vi "CH_LM FGV Meter Info.vi"(0 "Meter Index":i32, 2 "Action (read)":T4=enum."read", 5 "Serial Number (\"\")":string, 7 "Meter Info":T1, 11 "error in (no error)":errorcluster) -> (3 "All Meter Indices":i32[](array[numeric]), 4 "Meter Index out":i32, 6 "Serial Number out":string, 8 "Meter Info":T1, 13 "All Serial Numbers":string[](array[string]), 14 "All Meter Infos":T1[](array[typedef]), 15 "error out":errorcluster)   [LabVIEW 2017, in "CH_LM.lvlib"]
doc: "This VI is used as functional global variable and it stores LabMax meter indices and serial numbers with corresponding queue references in not initialized shift-registers.\n\nFour actions are supported: add, read, read by serial, set, remove and delete element (meter index, serial number, cluster of three queue references) and clear shift-registers.\n\nRemove element does not actually remove the element from the shift register but replaces the indexed element with default values.\n\n<B>Possible errors:</B>\n-1301: Serial number already existing.\n-1302: Serial number not found.\n-1306: Meter already existing.\n-1307: Meter index not found."
uses:
  CH_LM.lvlib
  CH_LM Meter Info.ctl
  _CH_LM/CH_LM Queue Cluster.ctl
  _CH_LM/CH_LM Event Cluster.ctl
  CH_LM Data Token.ctl
  _CH_LM/CH_LM Action Enumeration.ctl
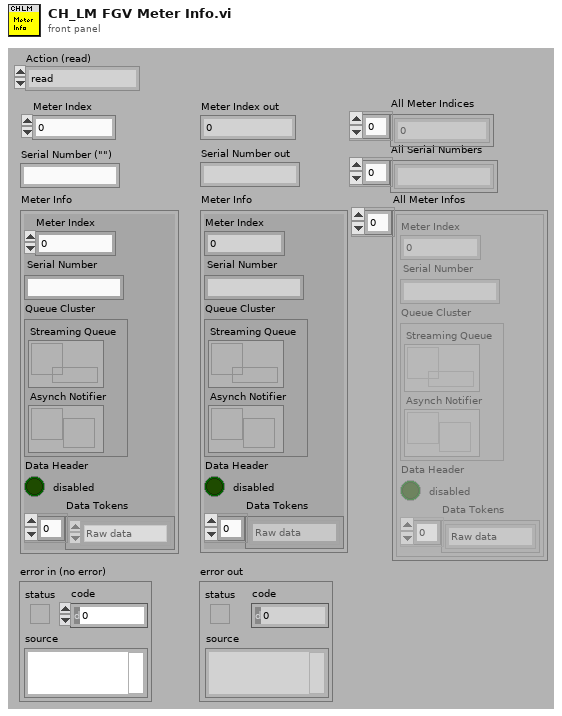
[diagram p1: front panel]
types:
  T1 = typedef "CH_LM.lvlib/CH_LM Meter Info.ctl" = cluster{"Meter Index":i32, "Serial Number":string, "Queue Cluster":T2, "Data Header":bool, "Data Tokens":T3[]}
  T2 = typedef "CH_LM.lvlib/CH_LM Queue Cluster.ctl" = cluster{"Streaming Queue":refnum<queue>, "Asynch Notifier":refnum<notifier>}
  T3 = typedef "CH_LM.lvlib/CH_LM Data Token.ctl" = enum16{"Raw data", "Quad distance", "Formated data", "Unit", "Pulse period", "Flags", "Sequence ID"}
  T4 = typedef "CH_LM.lvlib/CH_LM Action Enumeration.ctl" = enum16{"add", "read", "read by serial", "set", "remove", "delete", "Clear Shift-Register", ""}
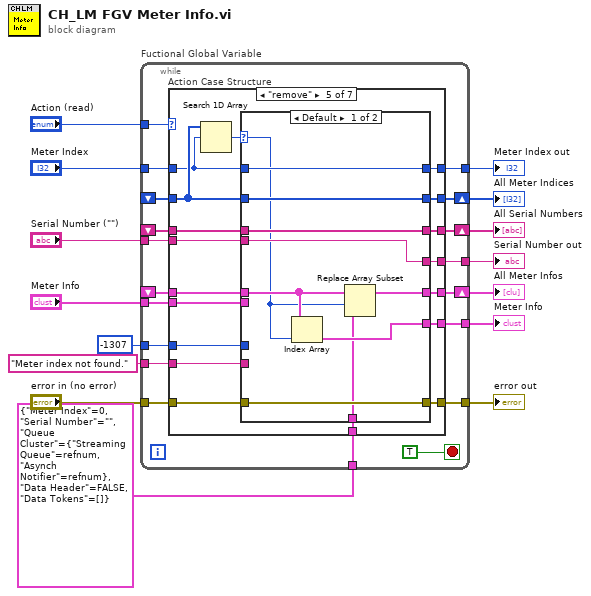
[diagram p0: block diagram]
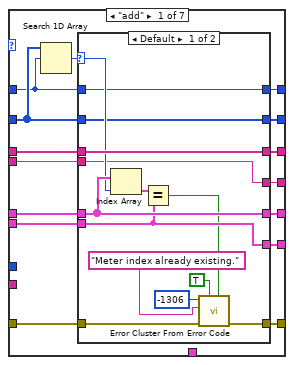
[diagram p2: hidden frame]
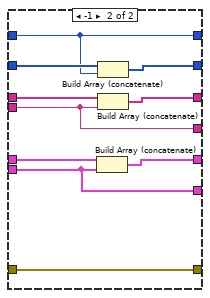
[diagram p3: hidden frame]
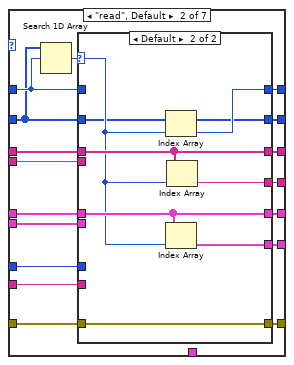
[diagram p4: hidden frame]
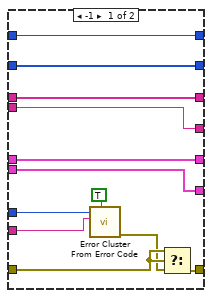
[diagram p5: hidden frame]
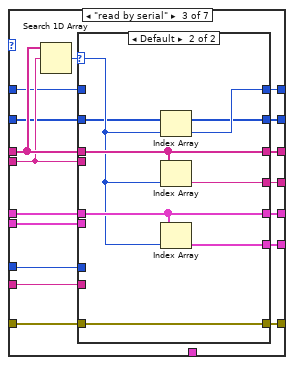
[diagram p6: hidden frame]
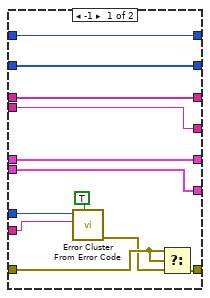
[diagram p7: hidden frame]
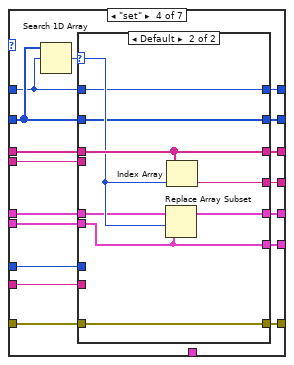
[diagram p8: hidden frame]
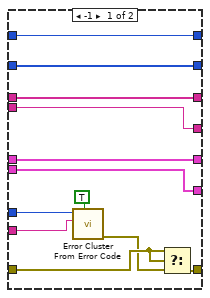
[diagram p9: hidden frame]
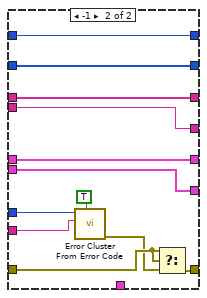
[diagram p10: hidden frame]
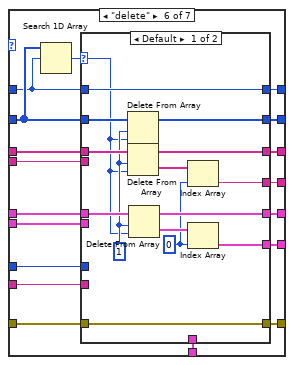
[diagram p11: hidden frame]
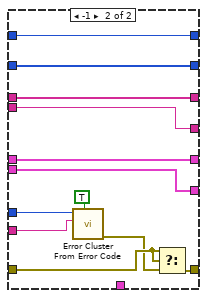
[diagram p12: hidden frame]
diagram:
  n1 = while "Fuctional Global Variable" {
    shift-right: [w26] -> w11
    shift-left: _ -> [w30]
    shift-right: [w25] -> w3
    shift-left: _ -> [w29]
    tunnel: "Action (read)" -> [w31]
    tunnel: "error in (no error)" -> [w33]
    tunnel: [w32] -> w14
    tunnel: "Serial Number (\"\")" -> [w28]
    tunnel: "Meter Info" -> [w27]
    tunnel: [w24] -> w10
    tunnel: [w23] -> w9
    shift-right: [w21] -> w6
    shift-left: _ -> [w20]
    tunnel: "Meter Index" -> [w22]
    tunnel: [w19] -> w5
    tunnel: T1 {"Meter Index"=0, "Serial Number"="", "Queue Cluster"={"Streaming Queue"=refnum, "Asynch Notifier"=refnum}, "Data Header"=FALSE, "Data Tokens"=[]} ("new element/subarray") -> [w18]
    tunnel: -1307 ("code") -> [w17]
    tunnel: "Meter index not found." -> [w16]
    stop <- TRUE stop-if-true
    n2 = case "Action Case Structure" shown="\"remove\"" w31 {
      tunnel: w33 -> [w44 w84 w121 w158 w196 w236 w271]
      tunnel: [w43 w83 w120 w157 w195 w235 w271] -> w32
      tunnel: w30 -> [w40 w86 w123 w160 w199 w239 _]
      tunnel: w29 -> [w49 w90 w127 w164 w203 w243 _]
      tunnel: w28 -> [w39 w80 w117 w154 w198 w238 _]
      tunnel: w27 -> [w48 w89 w126 w163 w202 w242 _]
      tunnel: [w47 w88 w125 w162 w201 w241 _] -> w26
      tunnel: [w46 w87 w124 w161 w200 w240 _] -> w25
      tunnel: [w42 w82 w119 w156 w194 w234 _] -> w24
      tunnel: [w41 w81 w118 w155 w193 w233 _] -> w23
      tunnel: w22 -> [w37 w78 w113 w150 w188 w228 _]
      tunnel: [w36 w79 w116 w153 w192 w232 _] -> w21
      tunnel: w20 -> [w38 w77 w115 w151 w189 w229 _]
      tunnel: [w35 w76 w114 w152 w191 w231 _] -> w19
      tunnel: w18 -> [_ _ _ _ w190 w230 _]
      tunnel: w17 -> [_ w75 w112 w149 w187 w227 _]
      tunnel: w16 -> [_ w74 w111 w148 w186 w226 _]
      frame "add" {
        n3 = Search 1D Array(1D array=w38, element=w37) -> (index of element=w45:i32)  [unwired: 1 out]
        n4 = case shown="Default" w45 {
          selector: w45 -> [w61 _]
          tunnel: w49 -> [w62 w73]
          tunnel: w48 -> [w59 w68]
          tunnel: [w63 w72] -> w47
          tunnel: [w62 w71] -> w46
          tunnel: w40 -> [w63 w70]
          tunnel: w39 -> [w58 w67]
          tunnel: w44 -> [w55 w69]
          tunnel: [w53 w69] -> w43
          tunnel: [w59 w68] -> w42
          tunnel: [w58 w67] -> w41
          tunnel: w38 -> [w57 w66]
          tunnel: w37 -> [w56 w64]
          tunnel: [w57 w65] -> w36
          tunnel: [w56 w64] -> w35
          frame Default {
            n5 = Index Array(array=w62, index=w61) -> (element=w60:T1)
            n6 = Equal?(x=w60, y=w59) -> (x = y?=w52:bool)
            n7 = call <vilib>:"Error Cluster From Error Code.vi"("is warning? (False)"=w52, "show call chain? (False)"=TRUE, "error in (no error)"=w55, "error message (\"\")"="Meter index already existing." ("error message (\"\")"), "error code (0)"=-1306) -> ("error out"=w53:errorcluster)  [unwired: 4 out]
          }
          frame -1 {
            n8 = Build Array (concatenate)(w73, w68) -> (w71:T1[])
            n9 = Build Array (concatenate)(w66, w64) -> (w65:i32[])
            n10 = Build Array (concatenate)(w70, w67) -> (w72:string[])
          }
        }
      }
      frame "read", Default {
        n11 = Search 1D Array(1D array=w77, element=w78) -> (index of element=w85:i32)  [unwired: 1 out]
        n12 = case shown="Default" w85 {
          selector: w85 -> [_ w105]
          tunnel: w90 -> [w101 w110]
          tunnel: w89 -> [w99 _]
          tunnel: [w102 w107] -> w88
          tunnel: [w101 w110] -> w87
          tunnel: w86 -> [w102 w107]
          tunnel: w84 -> [w95 w108]
          tunnel: [w100 w108] -> w83
          tunnel: [w99 w109] -> w82
          tunnel: [w98 w106] -> w81
          tunnel: w80 -> [w98 _]
          tunnel: w78 -> [w96 _]
          tunnel: [w97 w103] -> w79
          tunnel: w77 -> [w97 w103]
          tunnel: [w96 w104] -> w76
          tunnel: w75 -> [w92 _]
          tunnel: w74 -> [w91 _]
          frame -1 {
            n13 = call <vilib>:"Error Cluster From Error Code.vi"("show call chain? (False)"=TRUE, "error message (\"\")"=w91, "error code (0)"=w92) -> ("error out"=w94:errorcluster)  [unwired: 1 in, 5 out]
            n14 = Select(t=w95, s=w95, f=w94) -> (s? t:f=w100:errorcluster)
          }
          frame Default {
            n15 = Index Array(array=w103, index=w105) -> (element=w104:i32)
            n16 = Index Array(array=w110, index=w105) -> (element=w109:T1)
            n17 = Index Array(array=w107, index=w105) -> (element=w106:string)
          }
        }
      }
      frame "read by serial" {
        n18 = Search 1D Array(1D array=w123, element=w117) -> (index of element=w122:i32)  [unwired: 1 out]
        n19 = case shown="Default" w122 {
          selector: w122 -> [_ w142]
          tunnel: w127 -> [w138 w147]
          tunnel: w126 -> [w136 _]
          tunnel: [w139 w144] -> w125
          tunnel: [w138 w147] -> w124
          tunnel: w123 -> [w139 w144]
          tunnel: w121 -> [w135 w145]
          tunnel: [w137 w145] -> w120
          tunnel: [w136 w146] -> w119
          tunnel: [w134 w143] -> w118
          tunnel: w117 -> [w134 _]
          tunnel: [w133 w140] -> w116
          tunnel: w115 -> [w133 w140]
          tunnel: [w132 w141] -> w114
          tunnel: w113 -> [w132 _]
          tunnel: w112 -> [w129 _]
          tunnel: w111 -> [w128 _]
          frame -1 {
            n20 = call <vilib>:"Error Cluster From Error Code.vi"("show call chain? (False)"=TRUE, "error message (\"\")"=w128, "error code (0)"=w129) -> ("error out"=w130:errorcluster)  [unwired: 1 in, 5 out]
            n21 = Select(t=w135, s=w135, f=w130) -> (s? t:f=w137:errorcluster)
          }
          frame Default {
            n22 = Index Array(array=w140, index=w142) -> (element=w141:i32)
            n23 = Index Array(array=w144, index=w142) -> (element=w143:string)
            n24 = Index Array(array=w147, index=w142) -> (element=w146:T1)
          }
        }
      }
      frame "set" {
        n25 = Search 1D Array(1D array=w151, element=w150) -> (index of element=w159:i32)  [unwired: 1 out]
        n26 = case shown="Default" w159 {
          selector: w159 -> [_ w182]
          tunnel: w164 -> [w175 w179]
          tunnel: w163 -> [w173 w177]
          tunnel: [w176 w184] -> w162
          tunnel: [w175 w178] -> w161
          tunnel: w160 -> [w176 w184]
          tunnel: w158 -> [w172 w185]
          tunnel: [w174 w185] -> w157
          tunnel: [w173 w177] -> w156
          tunnel: [w171 w183] -> w155
          tunnel: w154 -> [w171 _]
          tunnel: [w170 w181] -> w153
          tunnel: w151 -> [w170 w181]
          tunnel: [w169 w180] -> w152
          tunnel: w150 -> [w169 w180]
          tunnel: w149 -> [w167 _]
          tunnel: w148 -> [w166 _]
          frame -1 {
            n27 = call <vilib>:"Error Cluster From Error Code.vi"("show call chain? (False)"=TRUE, "error message (\"\")"=w166, "error code (0)"=w167) -> ("error out"=w165:errorcluster)  [unwired: 1 in, 5 out]
            n28 = Select(t=w172, s=w172, f=w165) -> (s? t:f=w174:errorcluster)
          }
          frame Default {
            n29 = Replace Array Subset(array=w179, new element=w177, index=w182) -> (w178:T1[])
            n30 = Index Array(array=w184, index=w182) -> (element=w183:string)
          }
        }
      }
      frame "remove" {
        n31 = Search 1D Array(1D array=w189, element=w188) -> (index of element=w197:i32)  [unwired: 1 out]
        n32 = case shown="Default" w197 {
          selector: w197 -> [w206 _]
          tunnel: w203 -> [w207 w224]
          tunnel: w202 -> [_ w221]
          tunnel: [w209 w225] -> w201
          tunnel: [w212 w224] -> w200
          tunnel: w199 -> [w209 w225]
          tunnel: w198 -> [w208 w220]
          tunnel: w196 -> [w213 w222]
          tunnel: [w213 w223] -> w195
          tunnel: [w205 w221] -> w194
          tunnel: [w208 w220] -> w193
          tunnel: [w211 w219] -> w192
          tunnel: w189 -> [w211 w219]
          tunnel: [w210 w218] -> w191
          tunnel: w188 -> [w210 w218]
          tunnel: w190 -> [w204 _]
          tunnel: w187 -> [_ w216]
          tunnel: w186 -> [_ w215]
          frame Default {
            n33 = Index Array(array=w207, index=w206) -> (element=w205:T1)
            n34 = Replace Array Subset(array=w207, new element=w204, index=w206) -> (w212:T1[])
          }
          frame -1 {
            n35 = call <vilib>:"Error Cluster From Error Code.vi"("show call chain? (False)"=TRUE, "error message (\"\")"=w215, "error code (0)"=w216) -> ("error out"=w214:errorcluster)  [unwired: 1 in, 5 out]
            n36 = Select(t=w222, s=w222, f=w214) -> (s? t:f=w223:errorcluster)
          }
        }
      }
      frame "delete" {
        n37 = Search 1D Array(1D array=w229, element=w228) -> (index of element=w237:i32)  [unwired: 1 out]
        n38 = case shown="Default" w237 {
          selector: w237 -> [w249 _]
          tunnel: w243 -> [w255 w269]
          tunnel: w242 -> [_ w266]
          tunnel: [w251 w270] -> w241
          tunnel: [w257 w269] -> w240
          tunnel: w239 -> [w252 w270]
          tunnel: w238 -> [_ w265]
          tunnel: w236 -> [w258 w267]
          tunnel: [w258 w268] -> w235
          tunnel: [w245 w266] -> w234
          tunnel: [w247 w265] -> w233
          tunnel: [w253 w264] -> w232
          tunnel: w229 -> [w254 w264]
          tunnel: [w256 w263] -> w231
          tunnel: w228 -> [w256 w263]
          tunnel: w230 -> [_ _]
          tunnel: w227 -> [_ w261]
          tunnel: w226 -> [_ w260]
          frame Default {
            w244 = 0 ("index")
            w250 = 1 ("length")
            n39 = Delete From Array(array=w254, length=w250, index=w249) -> (array with subset deleted=w253:i32[])  [unwired: 1 out]
            n40 = Delete From Array(array=w252, length=w250, index=w249) -> (deleted portion=w248:string[], array with subset deleted=w251:string[])
            n41 = Delete From Array(array=w255, length=w250, index=w249) -> (deleted portion=w246:T1[], array with subset deleted=w257:T1[])
            n42 = Index Array(array=w248, index=w244) -> (element=w247:string)
            n43 = Index Array(array=w246, index=w244) -> (element=w245:T1)
          }
          frame -1 {
            n44 = call <vilib>:"Error Cluster From Error Code.vi"("show call chain? (False)"=TRUE, "error message (\"\")"=w260, "error code (0)"=w261) -> ("error out"=w259:errorcluster)  [unwired: 1 in, 5 out]
            n45 = Select(t=w267, s=w267, f=w259) -> (s? t:f=w268:errorcluster)
          }
        }
      }
      frame "Clear Shift-Register" {
      }
    }
  }
  "All Meter Infos" <- w3
  "All Serial Numbers" <- w11
  "Meter Info" <- w10
  "error out" <- w14
  "Serial Number out" <- w9
  "All Meter Indices" <- w6
  "Meter Index out" <- w5
